vi "DelayGeneratorSetOffset.vi"(8 "error in (no error)":errorcluster) -> (0 "error out":errorcluster)   [LabVIEW 2009]
uses:
  Controls/DelayTarget.ctl
panel:
  in  "Position":dbl[unit] format="%.6g"
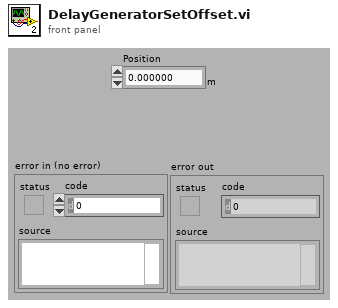
[diagram p1: front panel]
types:
  T1 = typedef "DelayTarget.ctl" = cluster{"Time":timestamp, "Position":dbl[unit], "Velocity":dbl[unit]}
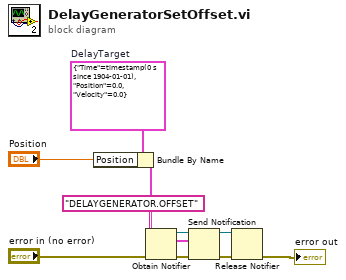
[diagram p0: block diagram]
diagram:
  w6 = T1 {"Time"=timestamp(0 s since 1904-01-01), "Position"=0.0, "Velocity"=0.0}  # DelayTarget
  n1 = Bundle By Name(cluster=w6, "Position"="Position") -> (w1:T1)
  n2 = Obtain Notifier(name (unnamed)="DELAYGENERATOR.OFFSET", notification data type=w1, error in (no error)="error in (no error)") -> (notifier out=w8:refnum<notifier>, error out=w7:errorcluster)  [unwired: 1 in, 1 out]
  n3 = Send Notification(notification=w1, notifier=w8, error in (no error)=w7) -> (notifier out=w2:refnum<notifier>, error out=w3:errorcluster)
  n4 = Release Notifier(notifier=w2, error in (no error)=w3) -> (error out=→"error out":errorcluster)  [unwired: 1 in, 2 out]
